vi "Pulse Gen Scan.vi"(8 "error in (no error)":errorcluster, 10 "Pulse Generator.lvclass":refnum<class "Pulse Generator.lvclass">, 11 "Pulse Gen Scan in":refnum<class "Pulse Gen Scan.lvclass">) -> (0 "error out":errorcluster, 3 "Pulse Gen Scan out":refnum<class "Pulse Gen Scan.lvclass">)   [LabVIEW 2009, in "Pulse Gen Scan.lvclass"]
uses:
  Pulse Gen Scan.lvclass
  Instruments/Pulse Gen/Pulse Generator.lvclass
  Scanner/Scanner.lvclass
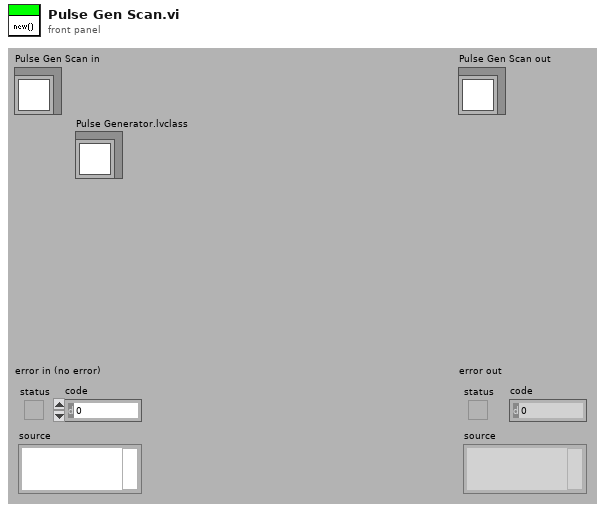
[diagram p1: front panel]
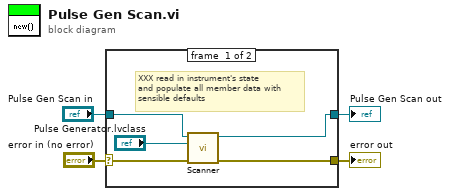
[diagram p0: block diagram]
diagram:
  n1 = case shown="No Error" "error in (no error)" {
    selector: "error in (no error)" -> [w9 w11]
    tunnel: [w7 w11] -> w3
    tunnel: [w6 w10] -> w1
    tunnel: "Pulse Gen Scan in" -> [w8 w10]
    frame #0 {
      # "XXX read in instrument's state\nand populate all member data with\nsensible defaults"
      n2 = call "Scanner.vi"("error in (no error)"=w9, "Scannable"="Pulse Generator.lvclass", "Scanner.lvclass in"=w8) -> ("error out"=w7:errorcluster, "Scanner.lvclass out"=w6:refnum<class "Pulse Gen Scan.lvclass">)  [unwired: 1 in, 6 out]
    }
    frame #1 {
    }
  }
  "error out" <- w3
  "Pulse Gen Scan out" <- w1
